vi "Serial Port Configure.vi"(5 "Parity (None)":enum32{"None", "Even", "Odd"}(ring), 6 "Flow Control (None)":enum32{"None", "Hardware"}(ring), 7 "Data Bits (8)":enum32{"7", "8"}(ring)=enum."8", 8 "error in (no error)":errorcluster, 9 "Baud Rate (9600)":T1(ring)=enum."9600", 10 "Node In":string, 11 "VISA resource name":refnum<visa-resource-name>) -> (0 "error out":errorcluster, 2 "Node Out":string, 3 "VISA resource name out":refnum<visa-resource-name>, 4 "Command String":string)   [LabVIEW 2018, in "Keithley 2600 Series.lvlib"]
doc: "This VI configures the instrument's RS-232 serial port.\n\n<b>Functions and Attributes Used</b>\nserial.baud\nserial.databits\nserial.flowcontrol\nserial.parity"
uses:
  Keithley 2600 Series.lvlib
  Private/GlobalVariables.vi
panel:
  # "(c) 2008 Keithley Instruments, Inc.  ALL RIGHTS RESERVED."
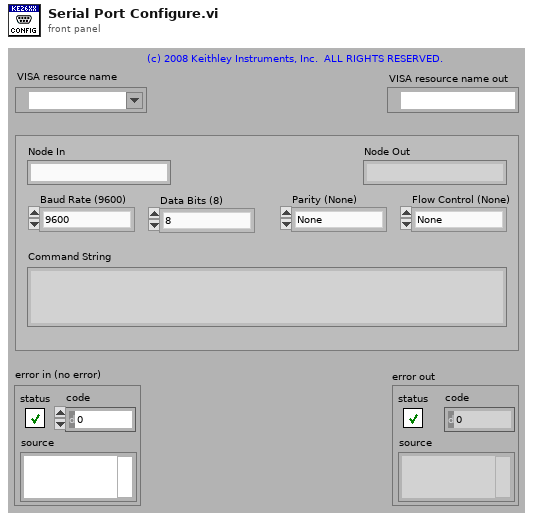
[diagram p1: front panel]
types:
  T1 = enum32{"300", "600", "1200", "2400", "4800", "9600", "19200", "38400", "57600", "115200"}
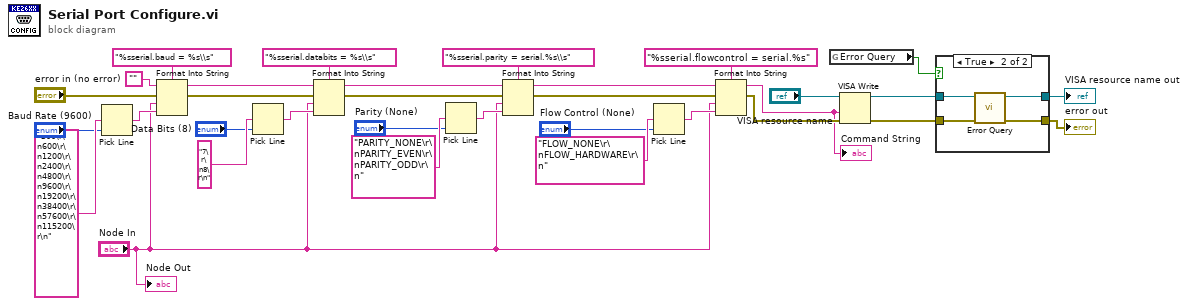
[diagram p0: block diagram]
diagram:
  n1 = Pick Line(multi-line string="300\r\n600\r\n1200\r\n2400\r\n4800\r\n9600\r\n19200\r\n38400\r\n57600\r\n115200\r\n" ("options"), line index="Baud Rate (9600)") -> (output string=w8:string)  [unwired: 1 out]
  n2 = Format Into String(format string="%sserial.baud = %s\\s", initial string="", error in="error in (no error)", "Node In", w8) -> (resulting string=w13:string, error out=w16:errorcluster)
  n3 = Pick Line(multi-line string="7\r\n8\r\n" ("options"), line index="Data Bits (8)") -> (output string=w7:string)  [unwired: 1 out]
  n4 = Format Into String(format string="%sserial.databits = %s\\s", initial string=w13, error in=w16, "Node In", w7) -> (resulting string=w12:string, error out=w15:errorcluster)
  n5 = Pick Line(multi-line string="PARITY_NONE\r\nPARITY_EVEN\r\nPARITY_ODD\r\n" ("options"), line index="Parity (None)") -> (output string=w6:string)  [unwired: 1 out]
  n6 = Format Into String(format string="%sserial.parity = serial.%s\\s", initial string=w12, error in=w15, "Node In", w6) -> (resulting string=w11:string, error out=w14:errorcluster)
  n7 = Pick Line(multi-line string="FLOW_NONE\r\nFLOW_HARDWARE\r\n" ("options"), line index="Flow Control (None)") -> (output string=w5:string)  [unwired: 1 out]
  n8 = Format Into String(format string="%sserial.flowcontrol = serial.%s", initial string=w11, error in=w14, "Node In", w5) -> (resulting string=w1:string, error out=w2:errorcluster)
  "Command String" <- w1
  n9 = global read "GlobalVariables.vi" "Error Query"() -> (w25:bool)
  n10 = VISA Write(VISA resource name="VISA resource name", write buffer=w1, error in (no error)=w2) -> (VISA resource name out=w24:refnum<visa-resource-name>, error out=w23:errorcluster)  [unwired: 1 out]
  n11 = case shown="True" w25 {
    tunnel: w24 -> [w35 w37]
    tunnel: w23 -> [w34 w39]
    tunnel: [w35 w36] -> w22
    tunnel: [w34 w38] -> w21
    frame False {
    }
    frame True {
      n12 = call "Error Query.vi"("error in (no error)"=w39, "VISA resource name"=w37) -> ("error out"=w38:errorcluster, "VISA resource name out"=w36:refnum<visa-resource-name>)  [unwired: 1 in, 7 out]
    }
  }
  "VISA resource name out" <- w22
  "error out" <- w21
  "Node Out" <- "Node In"
